vi "AssertTrue.vi"(7 "Message (\"\")":string, 8 "error in (no error)":errorcluster, 10 "Condition":bool) -> (0 "error out":errorcluster, 2 "Result":bool)   [LabVIEW 2019, in "Assertion.lvlib"]
doc: "Asserts that a condition is <B>true</B>. Does nothing if an error occurred before this node runs. Returns an error if the assertion failed. Optionally adds a message to the error message if the assertion failed."
uses:
  Assertion.lvlib
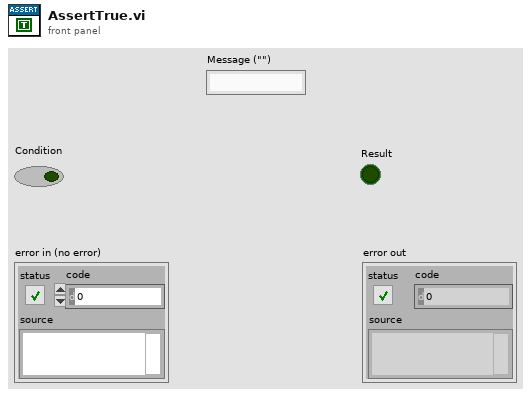
[diagram p1: front panel]
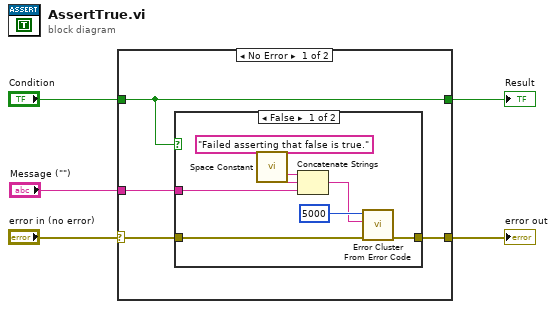
[diagram p0: block diagram]
diagram:
  n1 = case shown="No Error" "error in (no error)" {
    selector: "error in (no error)" -> [w8 w18]
    tunnel: [w9 _] -> w4
    tunnel: "Condition" -> [w9 _]
    tunnel: [w7 w18] -> w2
    tunnel: "Message (\"\")" -> [w6 _]
    frame No Error {
      n2 = case shown="False" w9 {
        tunnel: w8 -> [w16 w17]
        tunnel: [w15 w17] -> w7
        tunnel: w6 -> [w13 _]
        frame False {
          n3 = call <vilib>:"Space Constant.vi"() -> ("String"=w12:string)
          n4 = Concatenate Strings("Failed asserting that false is true.", w12, w13) -> (w10:string)
          n5 = call <vilib>:"Error Cluster From Error Code.vi"("error in (no error)"=w16, "error message (\"\")"=w10, "error code (0)"=5000) -> ("error out"=w15:errorcluster)  [unwired: 6 in]
        }
        frame True {
        }
      }
    }
    frame Error {
    }
  }
  "Result" <- w4
  "error out" <- w2
